vi "Create Point Style.vi"(4 "Cursor ID":i32, 5 "Sprite Type":T1, 7 "Size":sgl, 8 "error in (no error)":errorcluster, 9 "RGBA":cluster{"R":sgl, "G":sgl, "B":sgl, "A":sgl}, 10 "Scale":cluster{"X":sgl, "Y":sgl, "Z":sgl}, 11 "Position":cluster{"X":sgl, "Y":sgl, "Z":sgl}) -> (0 "error out":errorcluster, 3 "Scene:New Object":refnum<vi>)   [LabVIEW 2020, in "3D Plot.lvclass"]
uses:
  <vilib>/Math Plots/3D Math Plots/3D Plot/3D Plot/3D Plot.lvclass
  <vilib>/Math Plots/3D Math Plots/3D Plot/3D Plot/Typedef/Sprite Type.ctl
  <vilib>/picture/3D Picture Control/Object/Create Object (name).vi
  <vilib>/picture/3D Picture Control/NI_3D Picture Control.lvlib
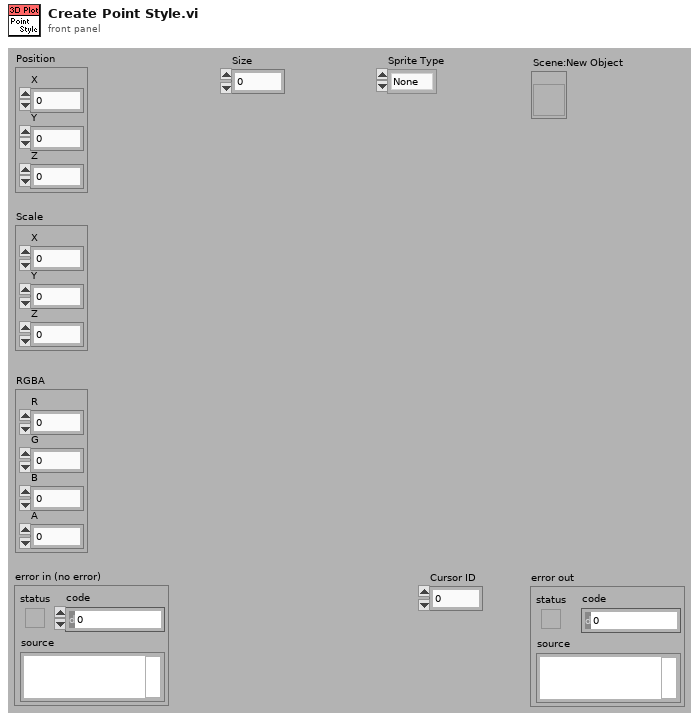
[diagram p1: front panel]
types:
  T1 = typedef "3D Plot.lvclass/Sprite Type.ctl" = enum16{"None", "Empty Square", "Solid Square", "Empty Diamond", "Solid Diamond", "Empty Circle", "Solid Circle", "Asterisk", "Bold X", "Wireframe Sphere", "Solid Sphere", "Wireframe Cube", "Solid Cube"}
  T2 = enum16{"Overall", "Per Primitive", "Per Vertex", "Binding Off"}
  T3 = enum16{"Points", "Lines", "Line Strip", "Line Loop", "Triangles", "Triangle Strip", "Triangle Fan", "Quads", "Quad Strip", "Polygon"}
  T4 = enum16{"Inherit Value", "Points", "Wireframe", "Polygons"}
  T5 = enum16{"Inherit Material", "Use entire Material", "Ignore Ambient", "Ignore Diffuse", "Ignore Specular", "Ignore Emission", "Ignore Ambient and Diffuse"}
  T6 = enum16{"Normal Bin", "Opaque Bin", "Transparent Bin"}
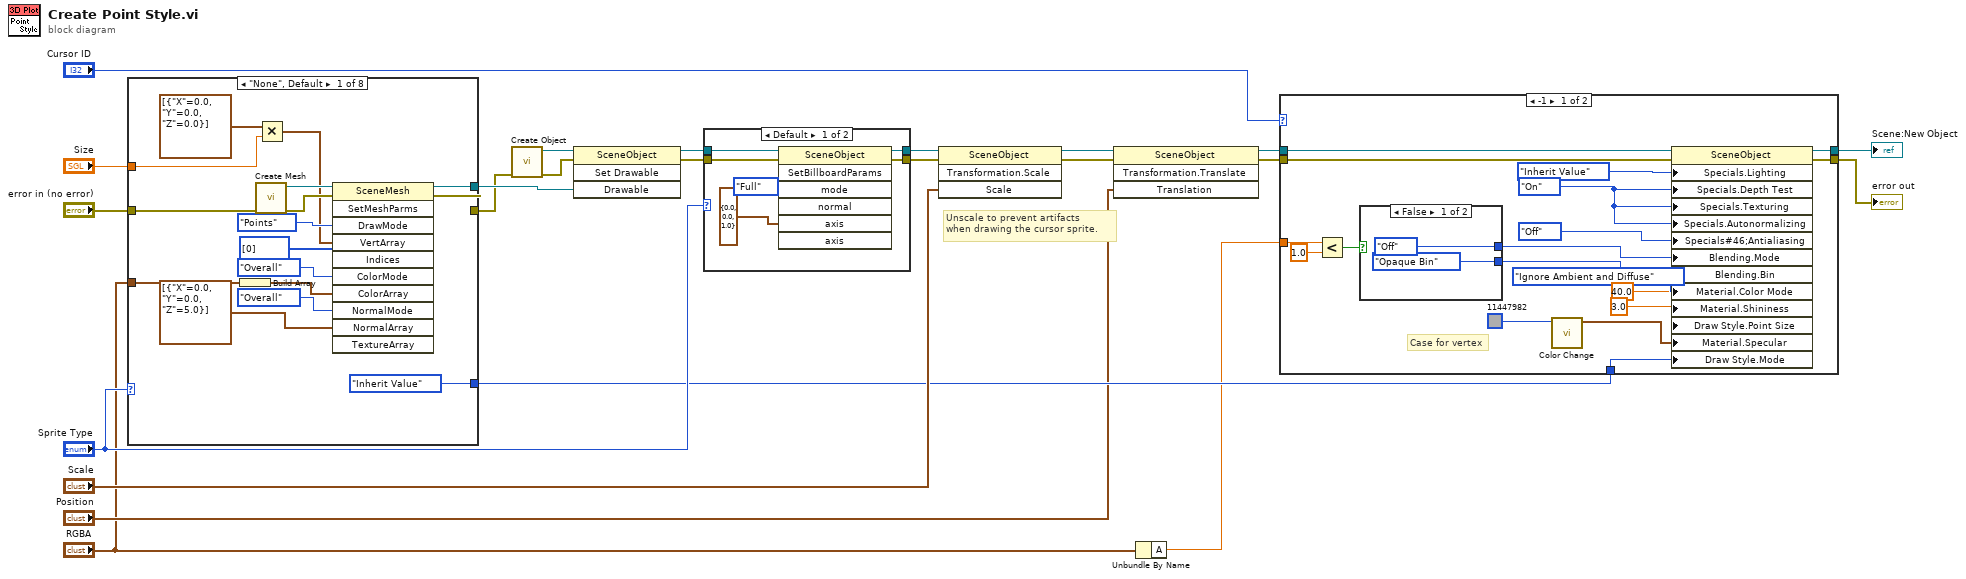
[diagram p0: block diagram]
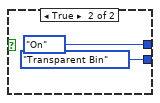
[diagram p2: hidden frame]
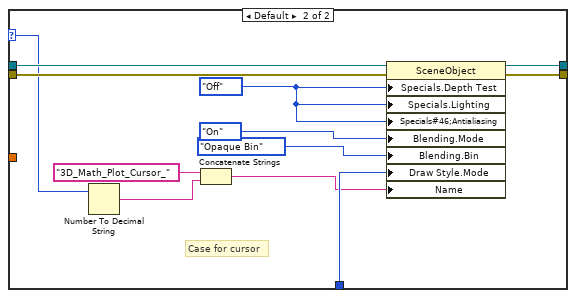
[diagram p3: hidden frame]
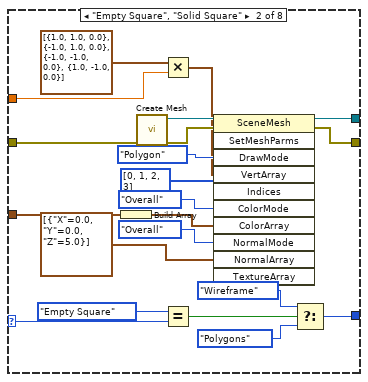
[diagram p5: hidden frame]
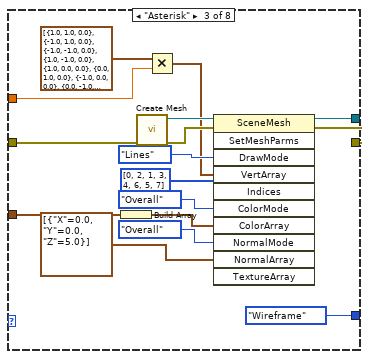
[diagram p6: hidden frame]
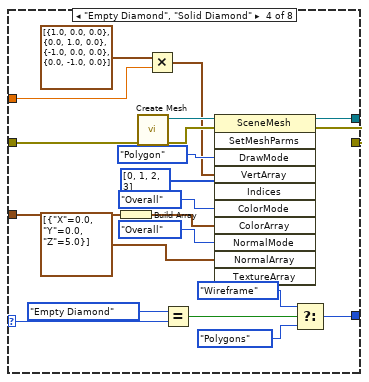
[diagram p7: hidden frame]
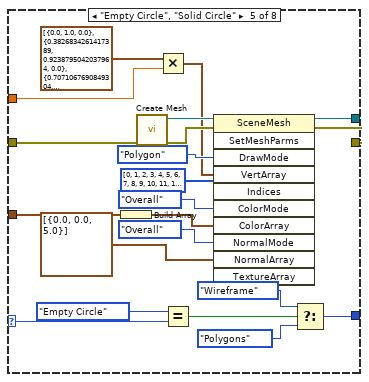
[diagram p8: hidden frame]
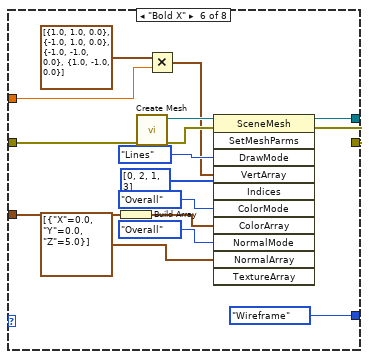
[diagram p9: hidden frame]
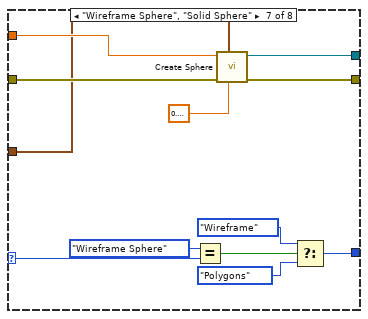
[diagram p10: hidden frame]
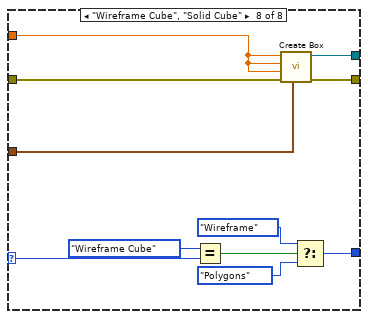
[diagram p11: hidden frame]
diagram:
  # "Unscale to prevent artifacts \nwhen drawing the cursor sprite."
  n1 = case shown="\"None\", Default" "Sprite Type" {
    selector: "Sprite Type" -> [_ w44 _ w80 w105 _ w136 w153]
    tunnel: "error in (no error)" -> [w29 w52 w69 w88 w106 w133 w146 w157]
    tunnel: [w27 w50 w68 w86 w103 w131 w145 w155] -> w10
    tunnel: "RGBA" -> [w24 w40 w61 w77 w98 w119 w135 w147]
    tunnel: "Size" -> [w30 w53 w70 w89 w107 w125 w144 w154]
    tunnel: [w28 w51 w67 w87 w102 w130 w143 w156] -> w14
    tunnel: [T4."Inherit Value" ("Draw Style:Mode") w45 T4."Wireframe" ("Draw Style:Mode") w81 w104 T4."Wireframe" ("Draw Style:Mode") w137 w149] -> w15
    frame "None", Default {
      n2 = Build Array(w24) -> (w33:cluster{"R":sgl, "G":sgl, "B":sgl, "A":sgl}[])
      n3 = call <vilib>:"Create Mesh.vi"("error in (no error)"=w29) -> ("error out"=w38:errorcluster, "New Mesh Refnum"=w39:refnum<vi>)  [unwired: 9 out]
      n4 = Multiply(x=cluster{"X":sgl, "Y":sgl, "Z":sgl}[] [{"X"=0.0, "Y"=0.0, "Z"=0.0}] ("Vertex Array"), y=w30) -> (x*y=w35:cluster{"X":sgl, "Y":sgl, "Z":sgl}[])
      n5 = invoke class="SceneMesh" method="SetMeshParms"(reference=w39, error in=w38, "DrawMode"=T3."Points" ("Draw Mode"), "VertArray"=w35, "Indices"=u32[] [0], "ColorMode"=T2."Overall" ("Color Binding Mode"), "ColorArray"=w33, "NormalMode"=T2."Overall" ("Normal Binding Mode"), "NormalArray"=cluster{"X":sgl, "Y":sgl, "Z":sgl}[] [{"X"=0.0, "Y"=0.0, "Z"=5.0}] ("Vertex Array")) -> (reference out=w28:refnum<vi>, error out=w27:errorcluster)  [unwired: 2 in, 9 out]
    }
    frame "Empty Square", "Solid Square" {
      n6 = Build Array(w40) -> (w54:cluster{"R":sgl, "G":sgl, "B":sgl, "A":sgl}[])
      n7 = call <vilib>:"Create Mesh.vi"("error in (no error)"=w52) -> ("error out"=w59:errorcluster, "New Mesh Refnum"=w60:refnum<vi>)  [unwired: 9 out]
      n8 = Multiply(x=cluster{"X":sgl, "Y":sgl, "Z":sgl}[] [{"X"=1.0, "Y"=1.0, "Z"=0.0}, {"X"=-1.0, "Y"=1.0, "Z"=0.0}, {"X"=-1.0, "Y"=-1.0, "Z"=0.0}, {"X"=1.0, "Y"=-1.0, "Z"=0.0}] ("Vertex Array"), y=w53) -> (x*y=w56:cluster{"X":sgl, "Y":sgl, "Z":sgl}[])
      n9 = Equal?(x=Sprite_Type."Empty Square" ("Sprite Type"), y=w44) -> (x = y?=w47:bool)
      n10 = invoke class="SceneMesh" method="SetMeshParms"(reference=w60, error in=w59, "DrawMode"=T3."Polygon" ("Draw Mode"), "VertArray"=w56, "Indices"=u32[] [0, 1, 2, 3], "ColorMode"=T2."Overall" ("Color Binding Mode"), "ColorArray"=w54, "NormalMode"=T2."Overall" ("Normal Binding Mode"), "NormalArray"=cluster{"X":sgl, "Y":sgl, "Z":sgl}[] [{"X"=0.0, "Y"=0.0, "Z"=5.0}] ("Vertex Array")) -> (reference out=w51:refnum<vi>, error out=w50:errorcluster)  [unwired: 2 in, 9 out]
      n11 = Select(t=T4."Wireframe" ("Draw Style:Mode"), s=w47, f=T4."Polygons" ("Draw Style:Mode")) -> (s? t:f=w45:T4)
    }
    frame "Asterisk" {
      n12 = Build Array(w61) -> (w71:cluster{"R":sgl, "G":sgl, "B":sgl, "A":sgl}[])
      n13 = call <vilib>:"Create Mesh.vi"("error in (no error)"=w69) -> ("error out"=w75:errorcluster, "New Mesh Refnum"=w76:refnum<vi>)  [unwired: 9 out]
      n14 = Multiply(x=cluster{"X":sgl, "Y":sgl, "Z":sgl}[] [{"X"=1.0, "Y"=1.0, "Z"=0.0}, {"X"=-1.0, "Y"=1.0, "Z"=0.0}, {"X"=-1.0, "Y"=-1.0, "Z"=0.0}, {"X"=1.0, "Y"=-1.0, "Z"=0.0}, {"X"=1.0, "Y"=0.0, "Z"=0.0}, {"X"=0.0, "Y"=1.0, "Z"=0.0}, {"X"=-1.0, "Y"=0.0, "Z"=0.0}, {"X"=0.0, "Y"=-1.0, "Z"=0.0}] ("Vertex Array"), y=w70) -> (x*y=w72:cluster{"X":sgl, "Y":sgl, "Z":sgl}[])
      n15 = invoke class="SceneMesh" method="SetMeshParms"(reference=w76, error in=w75, "DrawMode"=T3."Lines" ("Draw Mode"), "VertArray"=w72, "Indices"=u32[] [0, 2, 1, 3, 4, 6, 5, 7], "ColorMode"=T2."Overall" ("Color Binding Mode"), "ColorArray"=w71, "NormalMode"=T2."Overall" ("Normal Binding Mode"), "NormalArray"=cluster{"X":sgl, "Y":sgl, "Z":sgl}[] [{"X"=0.0, "Y"=0.0, "Z"=5.0}] ("Vertex Array")) -> (reference out=w67:refnum<vi>, error out=w68:errorcluster)  [unwired: 2 in, 9 out]
    }
    frame "Empty Diamond", "Solid Diamond" {
      n16 = Build Array(w77) -> (w90:cluster{"R":sgl, "G":sgl, "B":sgl, "A":sgl}[])
      n17 = call <vilib>:"Create Mesh.vi"("error in (no error)"=w88) -> ("error out"=w96:errorcluster, "New Mesh Refnum"=w97:refnum<vi>)  [unwired: 9 out]
      n18 = Multiply(x=cluster{"X":sgl, "Y":sgl, "Z":sgl}[] [{"X"=1.0, "Y"=0.0, "Z"=0.0}, {"X"=0.0, "Y"=1.0, "Z"=0.0}, {"X"=-1.0, "Y"=0.0, "Z"=0.0}, {"X"=0.0, "Y"=-1.0, "Z"=0.0}] ("Vertex Array"), y=w89) -> (x*y=w92:cluster{"X":sgl, "Y":sgl, "Z":sgl}[])
      n19 = Equal?(x=Sprite_Type."Empty Diamond" ("Sprite Type"), y=w80) -> (x = y?=w83:bool)
      n20 = invoke class="SceneMesh" method="SetMeshParms"(reference=w97, error in=w96, "DrawMode"=T3."Polygon" ("Draw Mode"), "VertArray"=w92, "Indices"=u32[] [0, 1, 2, 3], "ColorMode"=T2."Overall" ("Color Binding Mode"), "ColorArray"=w90, "NormalMode"=T2."Overall" ("Normal Binding Mode"), "NormalArray"=cluster{"X":sgl, "Y":sgl, "Z":sgl}[] [{"X"=0.0, "Y"=0.0, "Z"=5.0}] ("Vertex Array")) -> (reference out=w87:refnum<vi>, error out=w86:errorcluster)  [unwired: 2 in, 9 out]
      n21 = Select(t=T4."Wireframe" ("Draw Style:Mode"), s=w83, f=T4."Polygons" ("Draw Style:Mode")) -> (s? t:f=w81:T4)
    }
    frame "Empty Circle", "Solid Circle" {
      n22 = Build Array(w98) -> (w112:cluster{"R":sgl, "G":sgl, "B":sgl, "A":sgl}[])
      n23 = call <vilib>:"Create Mesh.vi"("error in (no error)"=w106) -> ("error out"=w117:errorcluster, "New Mesh Refnum"=w118:refnum<vi>)  [unwired: 9 out]
      n24 = Multiply(x=cluster{sgl, sgl, sgl}[] [{0.0, 1.0, 0.0}, {0.38268343, 0.9238795, 0.0}, {0.70710677, 0.70710677, 0.0}, {0.9238795, 0.38268343, 0.0}, {1.0, 6.123032e-17, 0.0}, {0.9238795, -0.38268343, 0.0}, {0.70710677, -0.70710677, 0.0}, {0.38268343, -0.9238795, 0.0}, {1.2246064e-16, -1.0, 0.0}, {-0.38268343, -0.9238795, 0.0}, {-0.70710677, -0.70710677, 0.0}, {-0.9238795, -0.38268343, 0.0}, {-1.0, -1.8369095e-16, 0.0}, {-0.9238795, 0.38268343, 0.0}, {-0.70710677, 0.70710677, 0.0}, {-0.38268343, 0.9238795, 0.0}] ("Array"), y=w107) -> (x*y=w114:cluster{sgl, sgl, sgl}[])
      n25 = Equal?(x=Sprite_Type."Empty Circle" ("Sprite Type"), y=w105) -> (x = y?=w109:bool)
      n26 = invoke class="SceneMesh" method="SetMeshParms"(reference=w118, error in=w117, "DrawMode"=T3."Polygon" ("Draw Mode"), "VertArray"=w114, "Indices"=u32[] [0, 1, 2, 3, 4, 5, 6, 7, 8, 9, 10, 11, 12, 13, 14, 15], "ColorMode"=T2."Overall" ("Color Binding Mode"), "ColorArray"=w112, "NormalMode"=T2."Overall" ("Normal Binding Mode"), "NormalArray"=cluster{sgl, sgl, sgl}[] [{0.0, 0.0, 5.0}] ("Array")) -> (reference out=w102:refnum<vi>, error out=w103:errorcluster)  [unwired: 2 in, 9 out]
      n27 = Select(t=T4."Wireframe" ("Draw Style:Mode"), s=w109, f=T4."Polygons" ("Draw Style:Mode")) -> (s? t:f=w104:T4)
    }
    frame "Bold X" {
      n28 = Build Array(w119) -> (w122:cluster{"R":sgl, "G":sgl, "B":sgl, "A":sgl}[])
      n29 = call <vilib>:"Create Mesh.vi"("error in (no error)"=w133) -> ("error out"=w132:errorcluster, "New Mesh Refnum"=w134:refnum<vi>)  [unwired: 9 out]
      n30 = Multiply(x=cluster{"X":sgl, "Y":sgl, "Z":sgl}[] [{"X"=1.0, "Y"=1.0, "Z"=0.0}, {"X"=-1.0, "Y"=1.0, "Z"=0.0}, {"X"=-1.0, "Y"=-1.0, "Z"=0.0}, {"X"=1.0, "Y"=-1.0, "Z"=0.0}] ("Vertex Array"), y=w125) -> (x*y=w124:cluster{"X":sgl, "Y":sgl, "Z":sgl}[])
      n31 = invoke class="SceneMesh" method="SetMeshParms"(reference=w134, error in=w132, "DrawMode"=T3."Lines" ("Draw Mode"), "VertArray"=w124, "Indices"=u32[] [0, 2, 1, 3], "ColorMode"=T2."Overall" ("Color Binding Mode"), "ColorArray"=w122, "NormalMode"=T2."Overall" ("Normal Binding Mode"), "NormalArray"=cluster{"X":sgl, "Y":sgl, "Z":sgl}[] [{"X"=0.0, "Y"=0.0, "Z"=5.0}] ("Vertex Array")) -> (reference out=w130:refnum<vi>, error out=w131:errorcluster)  [unwired: 2 in, 9 out]
    }
    frame "Wireframe Sphere", "Solid Sphere" {
      n32 = Equal?(x=Sprite_Type."Wireframe Sphere" ("Sprite Type"), y=w136) -> (x = y?=w139:bool)
      n33 = call <vilib>:"Create Sphere.vi"("Detail"=sgl 0.3, "Color"=w135, "error in (no error)"=w146, "Radius"=w144) -> ("error out"=w145:errorcluster, "New Sphere Refnum"=w143:refnum<vi>)  [unwired: 1 in, 5 out]
      n34 = Select(t=T4."Wireframe" ("Draw Style:Mode"), s=w139, f=T4."Polygons" ("Draw Style:Mode")) -> (s? t:f=w137:T4)
    }
    frame "Wireframe Cube", "Solid Cube" {
      n35 = Equal?(x=Sprite_Type."Wireframe Cube" ("Sprite Type"), y=w153) -> (x = y?=w150:bool)
      n36 = call <vilib>:"Create Box.vi"("Color"=w147, "error in (no error)"=w157, "Length Z"=w154, "Length Y"=w154, "Length X"=w154) -> ("error out"=w155:errorcluster, "New Box Refnum"=w156:refnum<vi>)  [unwired: 5 out]
      n37 = Select(t=T4."Wireframe" ("Draw Style:Mode"), s=w150, f=T4."Polygons" ("Draw Style:Mode")) -> (s? t:f=w149:T4)
    }
  }
  n38 = call-poly <vilib>:"Create Object.vi"("error in (no error)"=w10) -> ("error out"=w7:errorcluster, "Scene:New Object"=w8:refnum<vi>)  [unwired: 9 in]
  n39 = invoke class="SceneObject" method="Set Drawable"(reference=w8, error in=w7, "Drawable"=w14) -> (reference out=w16:refnum<vi>, error out=w17:errorcluster)  [unwired: 1 in, 2 out]
  n40 = case shown="Default" "Sprite Type" {
    tunnel: w16 -> [w162 w165]
    tunnel: w17 -> [w161 w164]
    tunnel: [w160 w165] -> w22
    tunnel: [w159 w164] -> w23
    frame Default {
      n41 = invoke class="SceneObject" method="SetBillboardParams"(reference=w162, error in=w161, "mode"=enum16{"No Billboarding", "Axial", "Full"}."Full", "axis"=cluster{"X":sgl, "Y":sgl, "Z":sgl} {"X"=0.0, "Y"=0.0, "Z"=1.0} ("normal")) -> (reference out=w160:refnum<vi>, error out=w159:errorcluster)  [unwired: 3 in, 5 out]
    }
    frame "Wireframe Sphere".."Solid Cube" {
    }
  }
  n42 = invoke class="SceneObject" method="Transformation.Scale"(reference=w22, error in=w23, "Scale"="Scale") -> (reference out=w21:refnum<vi>, error out=w20:errorcluster)  [unwired: 1 in, 2 out]
  n43 = invoke class="SceneObject" method="Transformation.Translate"(reference=w21, error in=w20, "Translation"="Position") -> (reference out=w11:refnum<vi>, error out=w12:errorcluster)  [unwired: 1 in, 2 out]
  n44 = Unbundle By Name("RGBA") -> ("A"=w1:sgl)
  n45 = case shown="-1" "Cursor ID" {
    selector: "Cursor ID" -> [_ w190]
    tunnel: w15 -> [w183 w195]
    tunnel: [w182 w196] -> w4
    tunnel: [w181 w197] -> w5
    tunnel: w12 -> [w180 w198]
    tunnel: w11 -> [w179 w199]
    tunnel: w1 -> [w166 _]
    frame -1 {
      w171 = enum16{"Inherit Value", "Off", "On"}."On" ("Specials:Depth Test")
      # "Case for vertex"
      n46 = Less?(x=w166, y=sgl 1.0) -> (x < y?=w169:bool)
      n47 = case shown="False" w169 {
        tunnel: [T6."Opaque Bin" ("Blending:Bin") T6."Transparent Bin" ("Blending:Bin")] -> w167
        tunnel: [enum16{"Inherit Value", "Off", "On"}."Off" ("Blending:Mode") enum16{"Inherit Value", "Off", "On"}."On" ("Blending:Mode")] -> w168
        frame False {
        }
        frame True {
        }
      }
      n48 = call <vilib>:"Color Change.vi"("Color"=u32 11447982) -> ("RGBA"=w172:cluster{"R":sgl, "G":sgl, "B":sgl, "A":sgl})  [unwired: 1 in, 9 out]
      n49 = property class="SceneObject"(reference=w179, error in=w180, "Specials.Lighting"=enum16{"Inherit Value", "Off", "On"}."Inherit Value" ("Specials:Lighting"), "Specials.Depth Test"=w171, "Specials.Texturing"=w171, "Specials.Autonormalizing"=w171, "Specials#46;Antialiasing"=enum16{"Inherit Value", "Off", "On"}."Off" ("Specials:Antialiasing"), "Blending.Mode"=w168, "Blending.Bin"=w167, "Material.Color Mode"=T5."Ignore Ambient and Diffuse" ("Material:Color Mode"), "Material.Shininess"=sgl 40.0 ("Material:Shininess"), "Draw Style.Point Size"=sgl 3.0 ("Draw Style:Point Size"), "Material.Specular"=w172, "Draw Style.Mode"=w183) -> (reference out=w181:refnum<vi>, error out=w182:errorcluster)
    }
    frame Default {
      w193 = enum16{"Inherit Value", "Off", "On"}."Off" ("Specials:Depth Test")
      # "Case for cursor"
      n50 = Number To Decimal String(number=w190) -> (decimal integer string=w189:string)  [unwired: 1 out]
      n51 = Concatenate Strings("3D_Math_Plot_Cursor_" ("string"), w189) -> (w188:string)
      n52 = property class="SceneObject"(reference=w199, error in=w198, "Specials.Depth Test"=w193, "Specials.Lighting"=w193, "Specials#46;Antialiasing"=w193, "Blending.Mode"=enum16{"Inherit Value", "Off", "On"}."On" ("Blending:Mode"), "Blending.Bin"=T6."Opaque Bin" ("Blending:Bin"), "Draw Style.Mode"=w195, "Name"=w188) -> (reference out=w197:refnum<vi>, error out=w196:errorcluster)
    }
  }
  "error out" <- w4
  "Scene:New Object" <- w5
